vi "Page Explorer - Tools Menu.vi"   [LabVIEW 2020]
types:
  T1 = enum32{"Invalid", "Standard", "Closed", "Hidden", "Minimized", "Maximized"}
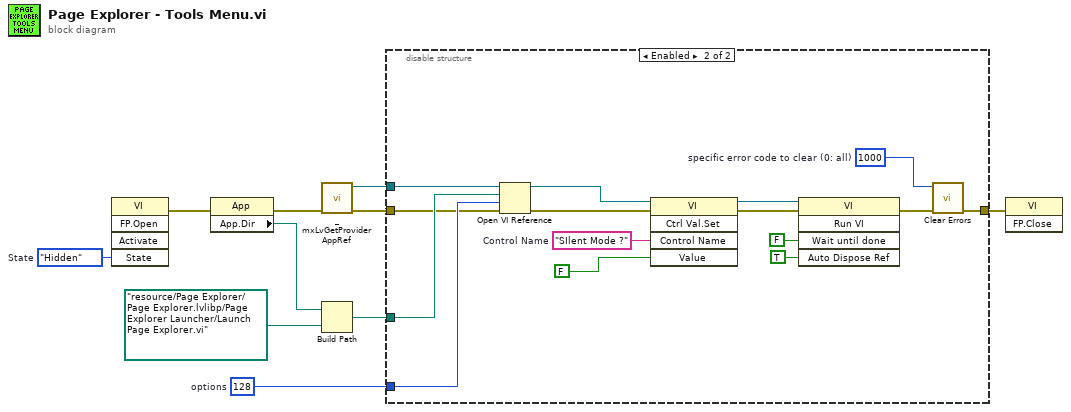
[diagram p0: block diagram]
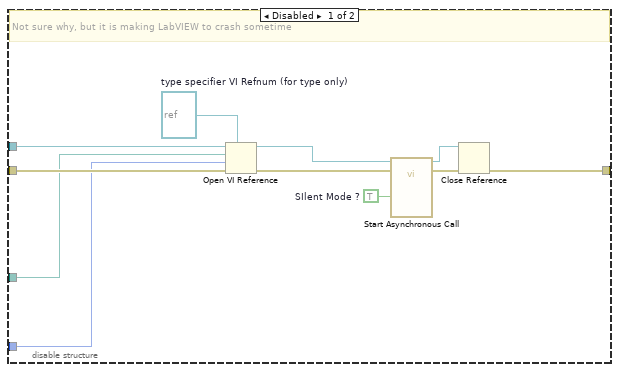
[diagram p2: hidden frame]
diagram:
  w2 = 128  # options
  w10 = T1."Hidden"  # State
  n1 = invoke class="VI" method="FP.Open"("State"=w10) -> (error out=w7:errorcluster)  [unwired: 4 in, 4 out]
  n2 = property class="App"(error in=w7) -> (error out=w6:errorcluster, "App.Dir"=w9:path)  [unwired: 1 in, 1 out]
  n3 = call "_mxLvGetProviderAppRef.vi"("error in"=w6) -> ("error out"=w5:errorcluster, "App Reference"=w4:refnum<vi>)  [unwired: 9 in]
  n4 = Build Path(base path=w9, name or relative path=path "resource/Page Explorer/Page Explorer.lvlibp/Page Explorer Launcher/Launch Page Explorer.vi" ("vi path")) -> (appended path=w3:path)
  n5 = disable-structure shown="Enabled" {
    disable-tunnel: w5 -> [w17 w25]
    disable-tunnel: [w19 w23] -> w1
    disable-tunnel: w2 -> [w11 w29]
    disable-tunnel: w3 -> [w12 w28]
    disable-tunnel: w4 -> [w13 w27]
    frame Disabled {
      w15 = refnum<vi> refnum  # type specifier VI Refnum (for type only)
      w20 = TRUE  # SIlent Mode ?
      # "Not sure why, but it is making LabVIEW to crash sometime"
      n6 = Open VI Reference(type specifier VI Refnum (for type only)=w15, application reference (local)=w13, vi path=w12, options=w11, error in (no error)=w17) -> (vi reference=w14:refnum<vi>, error out=w16:errorcluster)  [unwired: 1 in]
      n7 = call-by-ref "Start Asynchronous Call"(reference=w14, error in=w16, "SIlent Mode ?"=w20) -> (reference out=w18:refnum<vi>, error out=w21:errorcluster)
      n8 = Close Reference(reference=w18, error in (no error)=w21) -> (error out=w19:errorcluster)
    }
    frame Enabled {
      w22 = 1000  # specific error code to clear (0: all)
      w31 = "SIlent Mode ?"  # Control Name
      n9 = Open VI Reference(application reference (local)=w27, vi path=w28, options=w29, error in (no error)=w25) -> (vi reference=w26:refnum<vi>, error out=w24:errorcluster)  [unwired: 2 in]
      n10 = invoke class="VI" method="Ctrl Val.Set"(reference=w26, error in=w24, "Control Name"=w31, "Value"=FALSE ("Auto Dispose Reference")) -> (reference out=w32:refnum<vi>, error out=w33:errorcluster)  [unwired: 1 in, 3 out]
      n11 = invoke class="VI" method="Run VI"(reference=w32, error in=w33, "Wait until done"=FALSE ("Wait Until Done"), "Auto Dispose Ref"=TRUE ("Auto Dispose Reference")) -> (error out=w34:errorcluster)  [unwired: 1 in, 4 out]
      n12 = call <vilib>:"Clear Errors.vi"("error in (no error)"=w34, "specific error code to clear (0: all)"=w22) -> ("error out"=w23:errorcluster)  [unwired: 4 in, 1 out]
    }
  }
  n13 = invoke class="VI" method="FP.Close"(error in=w1) -> ()  [unwired: 2 in, 3 out]
